vi "add_light-dark_jv_to_queue.vi"(9 "Measuring all pixels on cell?":bool, 10 "Scan settings array":T3[](array[typedef]) {"Settling delay (s)" min=0.0; "J-t illumination" items=["Light only", "Dark only", "Light then dark", "Dark then light"]; "Measurement speed" items=["Fast", "Normal", "High accuracy"]; "Illumination" items=["Light only", "Dark only", "Light then dark", "Dark then light"]; "Only repeat for best pixel" items=["only for best pixel", "for best 2 pixels", "for best 3 pixels", "for best 4 pixels", "for best 5 pixels", "for best 6 pixels", "for best 7 pixels", "for all pixels"]; "No. of repeat scans" min=1.0 step=1.0; "Max power best pixel only" items=["only the best pixel", "the best 2 pixels", "the best 3 pixels", "the best 4 pixels", "the best 5 pixels", "the best 6 pixels", "the best 7 pixels", "all pixels"]; "J-t best pixel only" items=["only the best pixel", "the best 2 pixels", "the best 3 pixels", "the best 4 pixels", "the best 5 pixels", "the best 6 pixels", "the best 7 pixels", "all pixels"]; "J-t measurement speed" items=["Fast", "Normal", "High Accuracy"]; "Stabilisation mode" items=["V", "I"]; "Measurement delay (ms)" min=10.0}, 11 "Cell settings cluster":T2) -> (3 "Light/dark array":T1(array[cluster]))   [LabVIEW 2016]
uses:
  TypeDefs/scan_settings.ctl
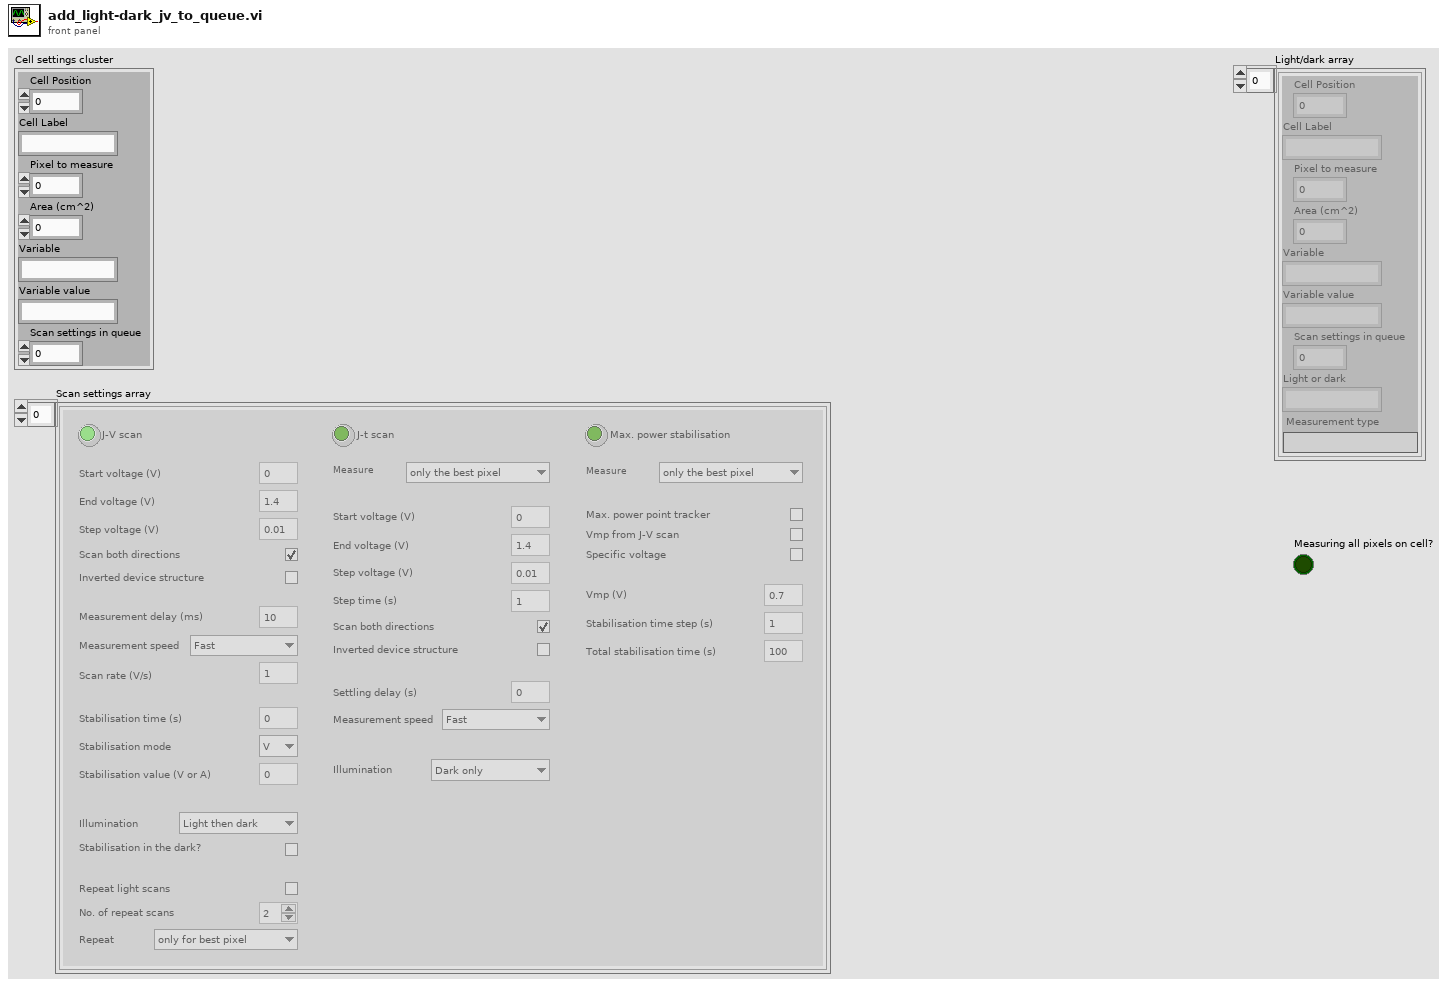
[diagram p1: front panel]
types:
  T1 = cluster{"Cell Position":i32, "Cell Label":string, "Pixel to measure":u16, "Area (cm^2)":dbl, "Variable":string, "Variable value":string, "Scan settings in queue":u16, "Light or dark":string, "Measurement type":string}[]
  T2 = cluster{"Cell Position":i32, "Cell Label":string, "Pixel to measure":u16, "Area (cm^2)":dbl, "Variable":string, "Variable value":string, "Scan settings in queue":u16}
  T3 = typedef "scan_settings.ctl" = cluster{"J-V scan":bool, "Start voltage (V)":dbl, "End voltage (V)":dbl, "Step voltage (V)":dbl, "Scan both directions":bool, "Inverted device structure":bool, "Measurement delay (ms)":dbl, "Measurement speed":u8, "Scan rate (V/s)":dbl, "Stabilisation time (s)":dbl, "Stabilisation mode":u16, "Stabilisation value (V or A) ":dbl, "Illumination":u16, "Stabilisation in the dark?":bool, "Repeat light scans":bool, "No. of repeat scans":dbl, "Only repeat for best pixel":u16, "J-t scan":bool, "J-t best pixel only":u16, "J-t start voltage (V)":dbl, "J-t end voltage (V)":dbl, "J-t step voltage (V)":dbl, "Step time (s)":dbl, "J-t scan both directions":bool, "J-t inverted device structure":bool, "Settling delay (s)":dbl, "J-t measurement speed":u16, "J-t illumination":u16, "Max. power stabilisation":bool, "Max power best pixel only":u16, "Max. power point tracker":bool, "Vmp from J-V scan":bool, "Max P stab. Specific voltage":bool, "Vmp (V)":dbl, "Stabilisation time step (s)":dbl, "Total stabilisation time (s)":dbl}
  T4 = cluster{"Cell Position":i32, "Cell Label":string, "Pixel to measure":u16, "Area (cm^2)":dbl, "Variable":string, "Variable value":string, "Scan settings in queue":u16, "Light or dark":string, "Measurement type":string}
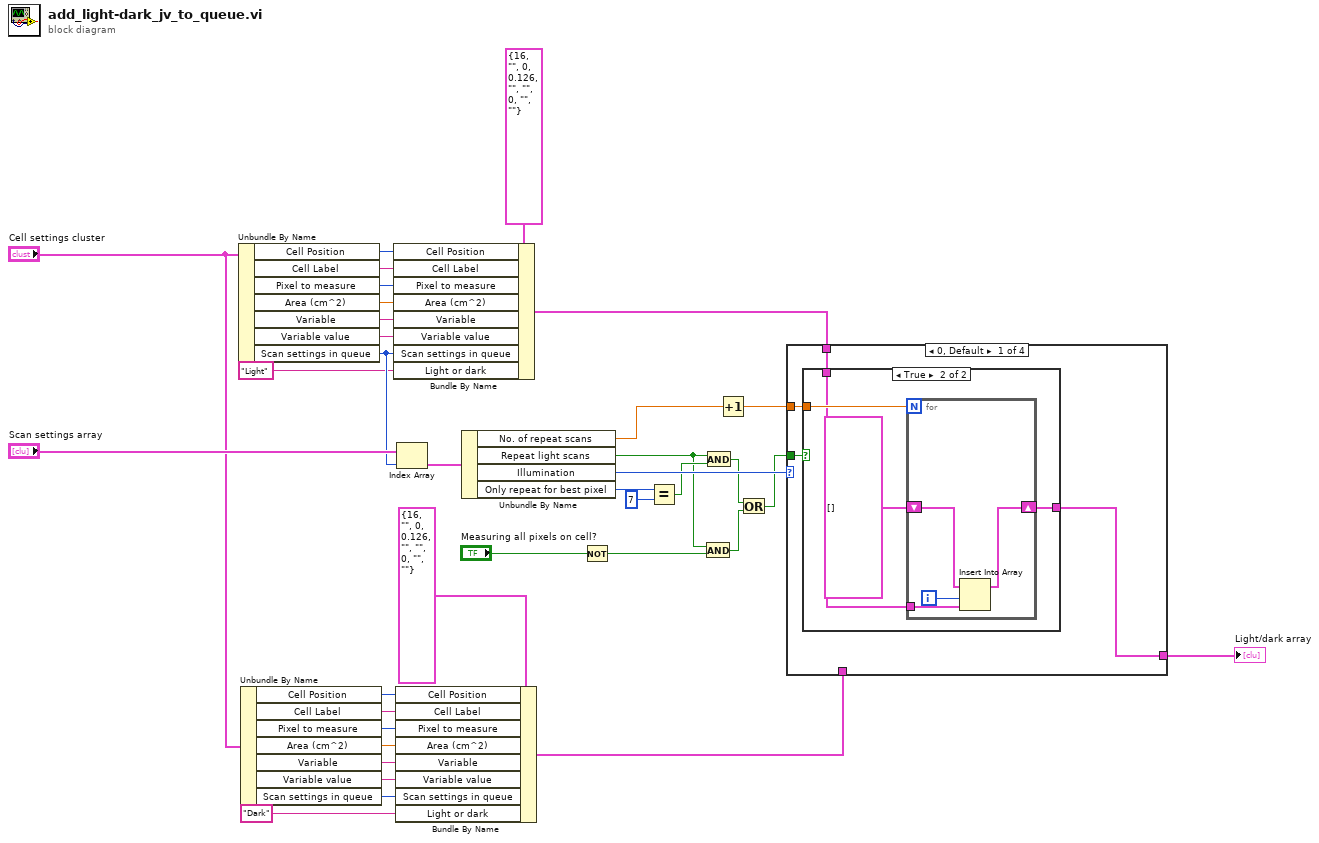
[diagram p0: block diagram]
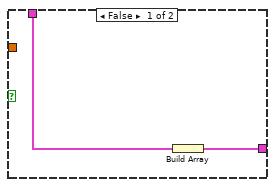
[diagram p2: hidden frame]
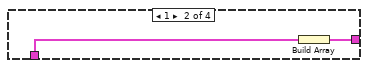
[diagram p3: hidden frame]
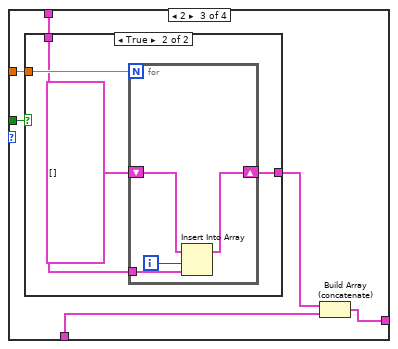
[diagram p4: hidden frame]
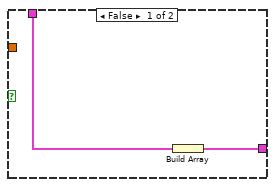
[diagram p5: hidden frame]
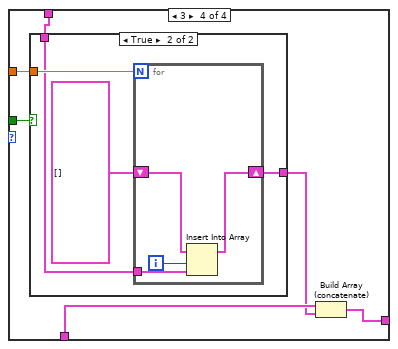
[diagram p6: hidden frame]
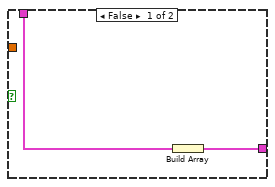
[diagram p7: hidden frame]
diagram:
  n1 = Unbundle By Name("Cell settings cluster") -> ("Cell Position"=w16:i32, "Cell Label"=w17:string, "Pixel to measure"=w18:u16, "Area (cm^2)"=w19:dbl, "Variable"=w20:string, "Variable value"=w21:string, "Scan settings in queue"=w34:u16)
  n2 = Unbundle By Name("Cell settings cluster") -> ("Cell Position"=w23:i32, "Cell Label"=w24:string, "Pixel to measure"=w25:u16, "Area (cm^2)"=w26:dbl, "Variable"=w27:string, "Variable value"=w28:string, "Scan settings in queue"=w29:u16)
  n3 = Bundle By Name(cluster=T4 {"Cell Position"=16, "Cell Label"="", "Pixel to measure"=0, "Area (cm^2)"=0.126, "Variable"="", "Variable value"="", "Scan settings in queue"=0, "Light or dark"="", "Measurement type"=""} ("System Cluster"), "Cell Position"=w16, "Cell Label"=w17, "Pixel to measure"=w18, "Area (cm^2)"=w19, "Variable"=w20, "Variable value"=w21, "Scan settings in queue"=w34, "Light or dark"="Light") -> (w14:T4)
  n4 = Bundle By Name(cluster=T4 {"Cell Position"=16, "Cell Label"="", "Pixel to measure"=0, "Area (cm^2)"=0.126, "Variable"="", "Variable value"="", "Scan settings in queue"=0, "Light or dark"="", "Measurement type"=""} ("System Cluster"), "Cell Position"=w23, "Cell Label"=w24, "Pixel to measure"=w25, "Area (cm^2)"=w26, "Variable"=w27, "Variable value"=w28, "Scan settings in queue"=w29, "Light or dark"="Dark") -> (w31:T4)
  n5 = Index Array(array="Scan settings array", index=w34) -> (element=w36:T3)
  n6 = Unbundle By Name(w36) -> ("No. of repeat scans"=w1:dbl, "Repeat light scans"=w8:bool, "Illumination"=w12:u16, "Only repeat for best pixel"=w11:u16)
  n7 = Not(x="Measuring all pixels on cell?") -> (.not. x?=w3:bool)
  n8 = Equal?(x=w11, y=u16 7) -> (x = y?=w9:bool)
  n9 = And(x=w8, y=w3) -> (x .and. y?=w7:bool)
  n10 = And(x=w8, y=w9) -> (x .and. y?=w6:bool)
  n11 = Increment(x=w1) -> (x+1=w2:dbl)
  n12 = Or(x=w6, y=w7) -> (x .or. y?=w5:bool)
  n13 = case shown="0, Default" w12 {
    tunnel: w14 -> [w38 _ w58 w72]
    tunnel: w31 -> [_ w52 w54 w74]
    tunnel: [w37 w51 w53 w73] -> w32
    tunnel: w5 -> [w39 _ w56 w70]
    tunnel: w2 -> [w40 _ w57 w71]
    frame 0, Default {
      n14 = case shown="True" w39 {
        tunnel: w40 -> [_ w46]
        tunnel: w38 -> [w42 w45]
        tunnel: [w41 w43] -> w37
        frame False {
          n15 = Build Array(w42) -> (w41:T1)
        }
        frame True {
          n16 = for {
            N: w46 -> [_]
            tunnel: w45 -> [w49]
            shift-right: [w47] -> w43
            shift-left: T1 [] ("Light/dark array") -> [w48]
            i -> [w50]
            n17 = Insert Into Array(array=w48, index=w50, new element=w49) -> (w47:T1)
          }
        }
      }
    }
    frame 1 {
      n18 = Build Array(w52) -> (w51:T1)
    }
    frame 2 {
      n19 = case shown="True" w56 {
        tunnel: w57 -> [_ w64]
        tunnel: w58 -> [w60 w63]
        tunnel: [w59 w61] -> w55
        frame False {
          n20 = Build Array(w60) -> (w59:T1)
        }
        frame True {
          n21 = for {
            N: w64 -> [_]
            tunnel: w63 -> [w67]
            shift-right: [w65] -> w61
            shift-left: T1 [] ("Light/dark array") -> [w66]
            i -> [w68]
            n22 = Insert Into Array(array=w66, index=w68, new element=w67) -> (w65:T1)
          }
        }
      }
      n23 = Build Array (concatenate)(w55, w54) -> (w53:T1)
    }
    frame 3 {
      n24 = case shown="True" w70 {
        tunnel: w71 -> [_ w80]
        tunnel: w72 -> [w76 w79]
        tunnel: [w75 w77] -> w69
        frame False {
          n25 = Build Array(w76) -> (w75:T1)
        }
        frame True {
          n26 = for {
            N: w80 -> [_]
            tunnel: w79 -> [w83]
            shift-right: [w81] -> w77
            shift-left: T1 [] ("Light/dark array") -> [w82]
            i -> [w84]
            n27 = Insert Into Array(array=w82, index=w84, new element=w83) -> (w81:T1)
          }
        }
      }
      n28 = Build Array (concatenate)(w74, w69) -> (w73:T1)
    }
  }
  "Light/dark array" <- w32
